vi "AerotechCloseSynchronization.vi"(2 "Synchro":T1, 9 "error in (no error)":errorcluster) -> (6 "error out":errorcluster)   [LabVIEW 2009]
uses:
  Controls/AerotechSynchro.ctl
  Controls/AerotechCommand.ctl
  Controls/AerotechState.ctl
  Controls/AerotechTarget.ctl
  Controls/AerotechScope.ctl
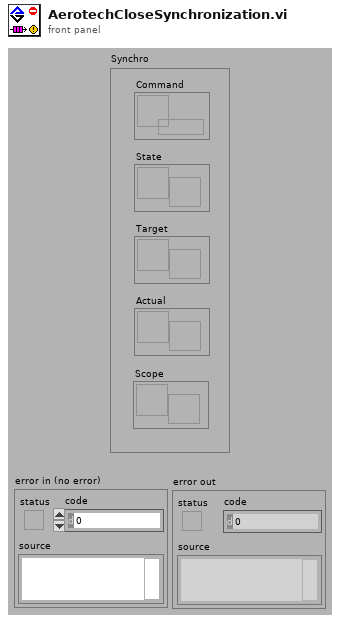
[diagram p1: front panel]
types:
  T1 = typedef "AerotechSynchro.ctl" = cluster{"Command":refnum<queue>, "State":refnum<notifier>, "Target":refnum<notifier>, "Actual":refnum<notifier>, "Scope":refnum<notifier>}
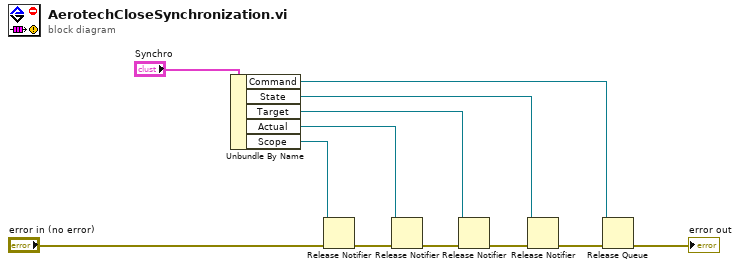
[diagram p0: block diagram]
diagram:
  n1 = Unbundle By Name("Synchro") -> ("Command"=w6:refnum<queue>, "State"=w7:refnum<notifier>, "Target"=w8:refnum<notifier>, "Actual"=w4:refnum<notifier>, "Scope"=w1:refnum<notifier>)
  n2 = Release Notifier(notifier=w1, error in (no error)="error in (no error)") -> (error out=w2:errorcluster)  [unwired: 1 in, 2 out]
  n3 = Release Notifier(notifier=w4, error in (no error)=w2) -> (error out=w5:errorcluster)  [unwired: 1 in, 2 out]
  n4 = Release Notifier(notifier=w8, error in (no error)=w5) -> (error out=w11:errorcluster)  [unwired: 1 in, 2 out]
  n5 = Release Notifier(notifier=w7, error in (no error)=w11) -> (error out=w10:errorcluster)  [unwired: 1 in, 2 out]
  n6 = Release Queue(queue=w6, error in (no error)=w10) -> (error out=→"error out":errorcluster)  [unwired: 1 in, 2 out]
